vi "Create Data Log.vi"(8 "error in (no error)":errorcluster, 10 "Test":string, 11 "Model in":refnum<class "Model.lvclass">) -> (0 "error out":errorcluster, 3 "Model out":refnum<class "Model.lvclass">)   [LabVIEW 2016, in "Model.lvclass"]
uses:
  Model.lvclass
  Typedefs/TestLogTypes.ctl
  Test Log/Test Log Factory/Test Log Factory.lvclass
  Model.lvclass/Model.ctl
  Test Log/Test Log/Test Log.lvclass
  Typedefs/HPMT_Typedefs.lvlib
panel:
  in  "error in (no error) 2":errorcluster
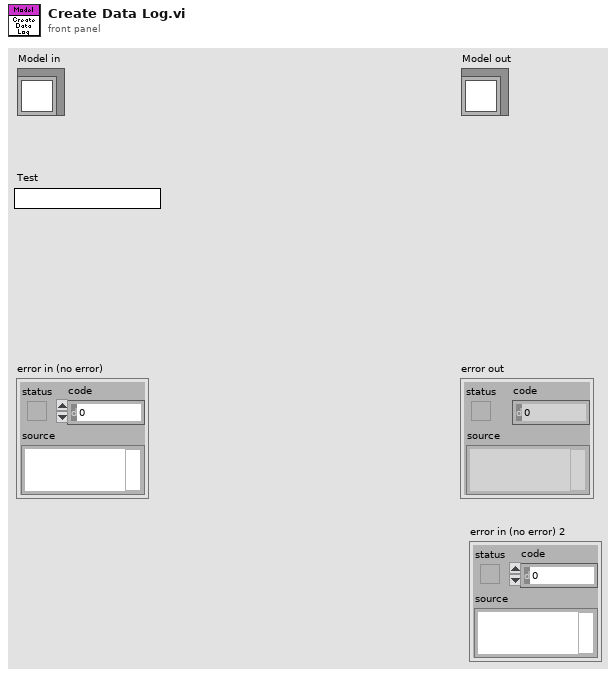
[diagram p1: front panel]
types:
  T1 = typedef "HPMT_Typedefs.lvlib/TestLogTypes.ctl" = enum16{"CSV Test Log"}
  T2 = typedef "HPMT_Typedefs.lvlib/TestSettings.ctl" = cluster{"Operator":string, "Actuator Serial Number":string, "Test Stand Serial Number":string, "Notes":string, "Load Cell Sensitivity":dbl}
  T3 = typedef "ActuatorData.ctl" = cluster{"Timestamp":dbl, "Force":dbl, "Encoder Value":i32}
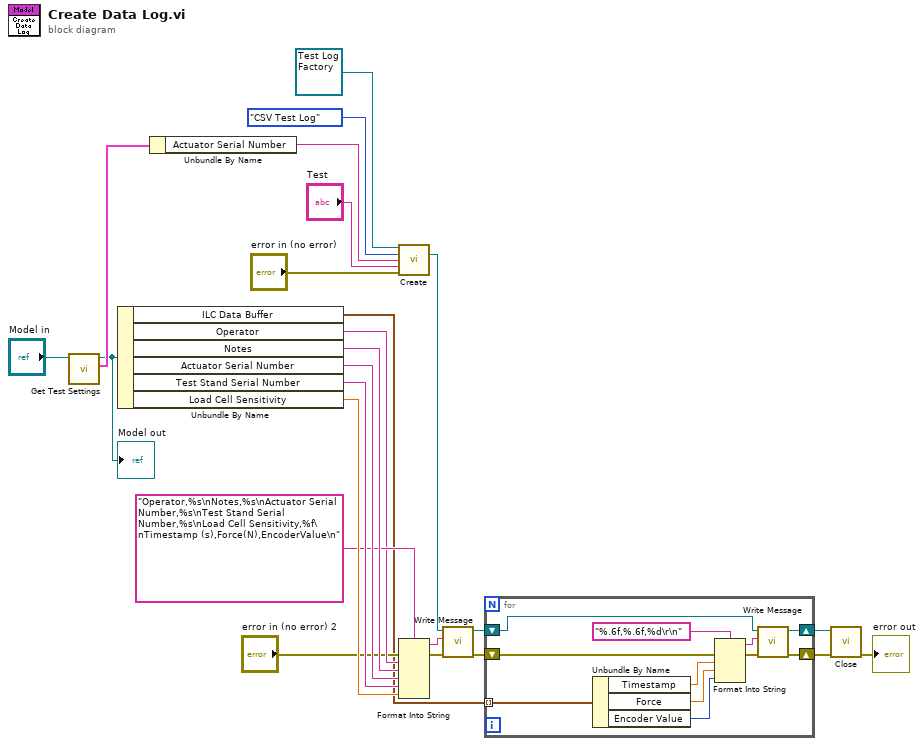
[diagram p0: block diagram]
diagram:
  n1 = call "Get Test Settings.vi"("Model in"="Model in") -> ("Test Settings"=w22:T2, "Model out"=w6:refnum<class "Model.lvclass">)  [unwired: 9 in]
  "Model out" <- w6
  n2 = Unbundle By Name(w6) -> ("ILC Data Buffer"=w2:T3[], "Operator"=w13:string, "Notes"=w15:string, "Actuator Serial Number"=w16:string, "Test Stand Serial Number"=w17:string, "Load Cell Sensitivity"=w18:dbl)
  n3 = Unbundle By Name(w22) -> ("Actuator Serial Number"=w24:string)
  n4 = call-dynamic "Create.vi"("Test Log Factory in"=refnum<class "Test Log Factory.lvclass"> refnum ("Test Log Factory.lvclass"), "Test Log Types"=TestLogTypes."CSV Test Log" ("TestLogTypes"), "Test Name"=w24, "Scan Name"="Test", "error in (no error)"="error in (no error)") -> ("Test Log"=w9:refnum<class "Test Log.lvclass">)  [unwired: 8 in, 2 out]
  n5 = Format Into String(format string="Operator,%s\nNotes,%s\nActuator Serial Number,%s\nTest Stand Serial Number,%s\nLoad Cell Sensitivity,%f\nTimestamp (s),Force(N),EncoderValue\n", error in="error in (no error) 2", w13, w15, w16, w17, w18) -> (resulting string=w10:string, error out=w11:errorcluster)  [unwired: 1 in]
  n6 = call-dynamic "Write Message.vi"("error in (no error)"=w11, "Message"=w10, "Test Log in"=w9) -> ("error out"=w3:errorcluster, "Test Log out"=w4:refnum<class "Test Log.lvclass">)  [unwired: 7 in]
  n7 = for {
    shift-right: [w33] -> w8
    shift-left: w4 -> [w34]
    shift-right: [w29] -> w7
    shift-left: w3 -> [w32]
    tunnel: w2 -> [w28] mode=indexing
    n8 = Unbundle By Name(w28) -> ("Timestamp"=w27:dbl, "Force"=w26:dbl, "Encoder Value"=w25:i32)
    n9 = Format Into String(format string="%.6f,%.6f,%d\r\n", error in=w32, w27, w26, w25) -> (resulting string=w30:string, error out=w31:errorcluster)  [unwired: 1 in]
    n10 = call-dynamic "Write Message.vi"("error in (no error)"=w31, "Message"=w30, "Test Log in"=w34) -> ("error out"=w29:errorcluster, "Test Log out"=w33:refnum<class "Test Log.lvclass">)  [unwired: 7 in]
  }
  n11 = call-dynamic "Close.vi"("error in (no error)"=w7, "Test Log in"=w8) -> ("error out"=→"error out":errorcluster)  [unwired: 8 in, 1 out]
